vi "Fwd Kenimatics - cluster.vi"(4 "To":i32=7, 7 "From":i32, 8 "Side":T1, 11 "Current":T2={"e0"=8.898926, "e1"=45.791016, "s0"=-1.252441, "s1"=-34.541016, "w0"=-12.875977, "w1"=74.750976, "w2"=9.008789} {"w2" scale=-175.25..175.25; "w1" scale=-90.0..120.0; "w0" scale=-175.25..175.25; "e1" scale=-3.0..150.0; "e0" scale=-173.5..173.5; "s1" scale=-123.0..60.0; "s0" scale=-141.0..51.0}) -> (0 "Matrix":T3 format="%.3f", 3 "Position":dbl[](array[numeric]) format="%.3f")   [LabVIEW 2013]
uses:
  <vilib>/Analysis/Matrix/Datatypes/RealMatrix.ctl
  ROS/Code/JointPositions.ctl
  ROS/Code/SubVIs/BaxterSide.ctl
  <vilib>/Analysis/Matrix/NI_Matrix.lvlib
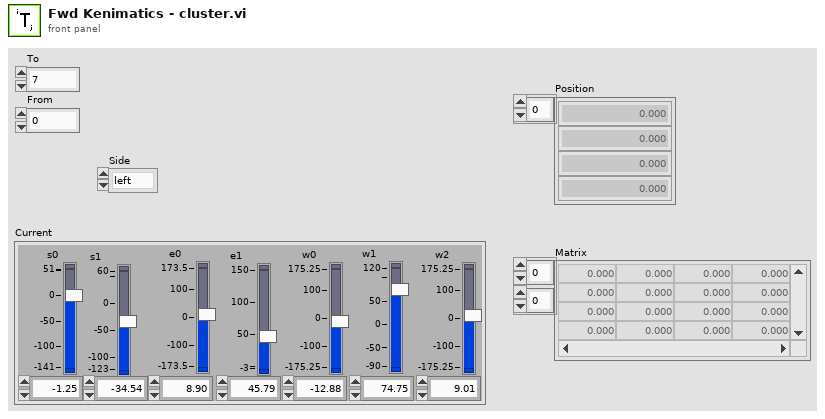
[diagram p1: front panel]
types:
  T1 = typedef "BaxterSide.ctl" = enum16{"left", "right"}
  T2 = typedef "JointPositions.ctl" = cluster{"e0":dbl, "e1":dbl, "s0":dbl, "s1":dbl, "w0":dbl, "w1":dbl, "w2":dbl}
  T3 = typedef "NI_Matrix.lvlib/RealMatrix.ctl" = dbl[][]
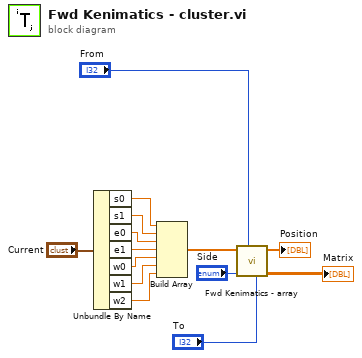
[diagram p0: block diagram]
diagram:
  n1 = Unbundle By Name("Current") -> ("s0"=w12:dbl, "s1"=w13:dbl, "e0"=w11:dbl, "e1"=w10:dbl, "w0"=w9:dbl, "w1"=w8:dbl, "w2"=w7:dbl)
  n2 = Build Array(w12, w13, w11, w10, w9, w8, w7) -> (w5:dbl[])
  n3 = call "Fwd Kenimatics - array.vi"("To"="To", "From"="From", "Side"="Side", "Joints"=w5) -> ("Matrix"=→"Matrix":T3, "Position"=→"Position":dbl[])  [unwired: 6 in]
